vi "ALTS-2015 Read Write ALTS INI Cluster.vi"(7 "Options":T2, 8 "error in (no error)":errorcluster, 10 "Configuration Cluster":T1, 11 "INI File Path":path=path "C:/Eaton/Audit Test System/Software/Info/EHMATS.ini") -> (0 "error out":errorcluster, 3 "Configuration Cluster Out":T1)   [LabVIEW 2013]
uses:
  Controls/ALTS-2015 LV2GBL Options.ctl
  Controls/ALTS-2015 INI Configuration Cluster.ctl
  <vilib>/Utility/config.llb/NI_LVConfig.lvlib
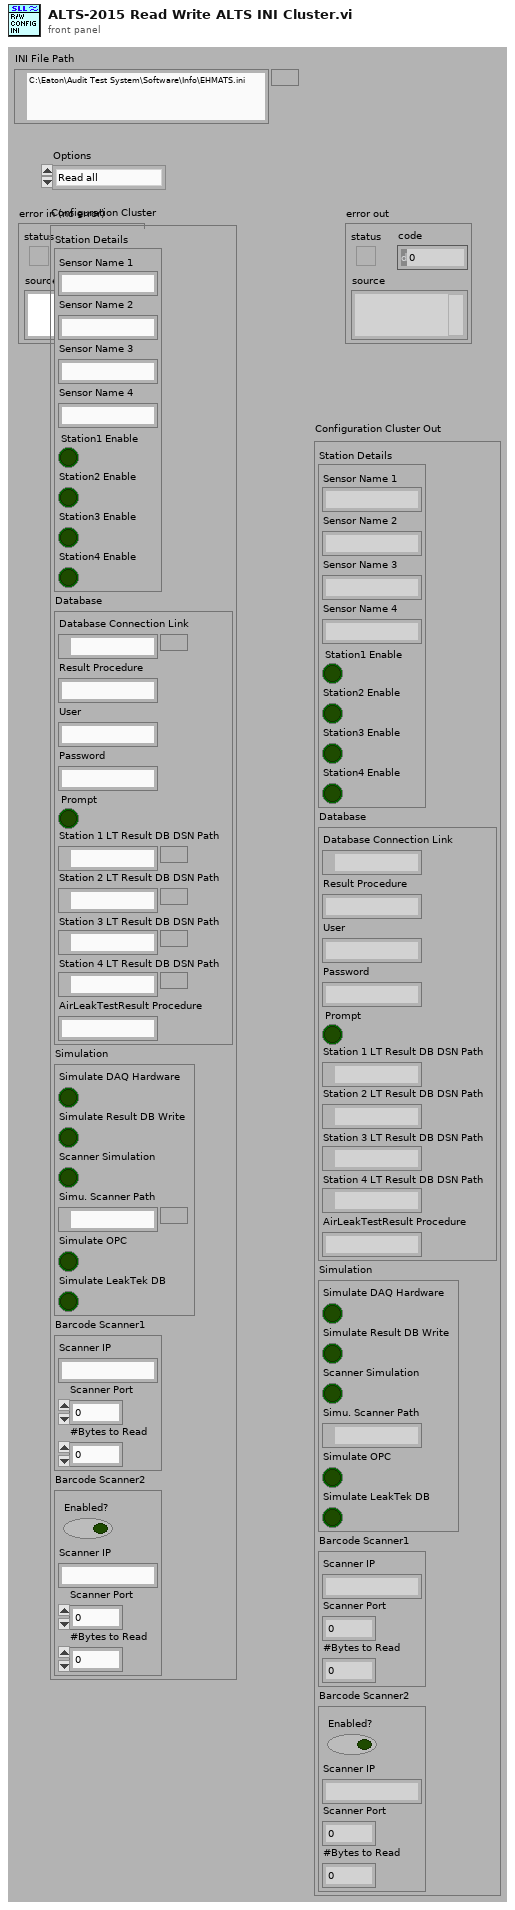
[diagram p1: front panel]
types:
  T1 = typedef "ALTS-2015 INI Configuration Cluster.ctl" = cluster{"Station Details":cluster{"Sensor Name 1":string, "Sensor Name 2":string, "Sensor Name 3":string, "Sensor Name 4":string, "Station1 Enable":bool, "Station2 Enable":bool, "Station3 Enable":bool, "Station4 Enable":bool}, "Database":cluster{"Database Connection Link":path, "Result Procedure":string, "User":string, "Password":string, "Prompt":bool, "Station 1 LT Result DB DSN Path":path, "Station 2 LT Result DB DSN Path":path, "Station 3 LT Result DB DSN Path":path, "Station 4 LT Result DB DSN Path":path, "AirLeakTestResult Procedure":string}, "Simulation":cluster{"Simulate DAQ Hardware":bool, "Simulate Result DB Write":bool, "Scanner Simulation":bool, "Simu. Scanner Path":path, "Simulate OPC":bool, "Simulate LeakTek DB":bool}, "Barcode Scanner1":cluster{"Scanner IP":string, "Scanner Port":u16, "#Bytes to Read":i32}, "Barcode Scanner2":cluster{"Enabled?":bool, "Scanner IP":string, "Scanner Port":u16, "#Bytes to Read":i32}}
  T2 = typedef "ALTS-2015 LV2GBL Options.ctl" = enum16{"Read all", "Write all"}
  T3 = typedef "NI_LVConfig.lvlib/Config Data RefNum.ctl" = refnum<k1>
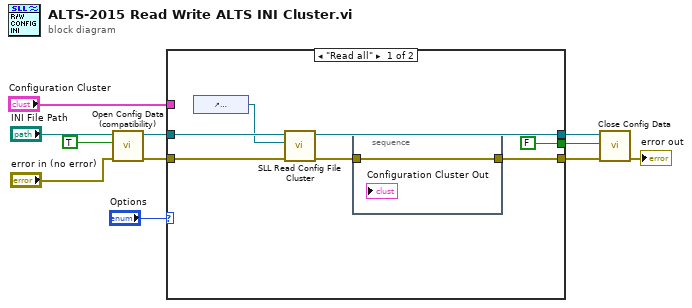
[diagram p0: block diagram]
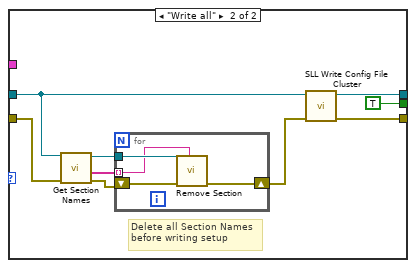
[diagram p2: hidden frame]
diagram:
  n1 = call <vilib>:"Open Config Data (compatibility).vi"("error in (no error)"="error in (no error)", "create file if necessary (T)"=TRUE ("create file if necessary? (T)"), "configuration file path"="INI File Path") -> ("error out"=w11:errorcluster, "refnum"=w10:T3)  [unwired: 6 in, 1 out]
  n2 = case shown="\"Read all\"" "Options" {
    tunnel: w11 -> [w17 w25]
    tunnel: w10 -> [w16 w23]
    tunnel: [w14 w21] -> w7
    tunnel: [w18 w24] -> w6
    tunnel: "Configuration Cluster" -> [_ _]
    tunnel: [FALSE ("write configuration file? (F)") TRUE ("write configuration file? (F)")] -> w2
    frame "Read all" {
      n3 = control-ref of="Configuration Cluster Out"() -> (w12:refnum<vi>)
      n4 = call <userlib>:"SLL Read Config File Cluster.vi"("error in (no error)"=w17, "Config File Cluster Refnum in"=w12, "Config File Refnum in"=w16) -> ("error out"=w15:errorcluster, "Config File Refnum out"=w18:T3)  [unwired: 7 in]
      n5 = stacked-sequence {
        tunnel: w15 -> [w19]
        tunnel: [w19] -> w14
        frame #0 {
        }
      }
    }
    frame "Write all" {
      # "Delete all Section Names\nbefore writing setup"
      n6 = call <vilib>:"Get Section Names.vi"("error in (no error)"=w25, "refnum"=w23) -> ("error out"=w26:errorcluster, "section names"=w28:string[], "refnum out"=w27:T3)  [unwired: 7 in]
      n7 = for {
        tunnel: w28 -> [w31] mode=indexing
        tunnel: w27 -> [w32]
        shift-right: [w29] -> w22
        shift-left: w26 -> [w30]
        n8 = call <vilib>:"Remove Section.vi"("section"=w31, "error in (no error)"=w30, "refnum"=w32) -> ("error out"=w29:errorcluster)  [unwired: 6 in, 2 out]
      }
      n9 = call <userlib>:"SLL Write Config File Cluster.vi"("error in (no error)"=w22, "Config File Refnum in"=w23) -> ("error out"=w21:errorcluster, "Config File Refnum out"=w24:T3)  [unwired: 8 in]
    }
  }
  n10 = call <vilib>:"Close Config Data.vi"("error in (no error)"=w7, "write file if changed (T)"=w2, "refnum"=w6) -> ("error out"=→"error out":errorcluster)  [unwired: 7 in, 1 out]
